vi "DatabaseView.vi"(11 "In_Database":string[][](array[string])) -> (3 "Out_Data":T1[](array[typedef]))   [LabVIEW 2020]
doc: "Na podstawie bazy danych, tworzy wizualizacjê wybieranych opcji przez w³aœciciela auta o danej tablicy rejestracyjnej."
uses:
  controls/BaseElemCluster.ctl
  controls/Car_wash_indicators.ctl
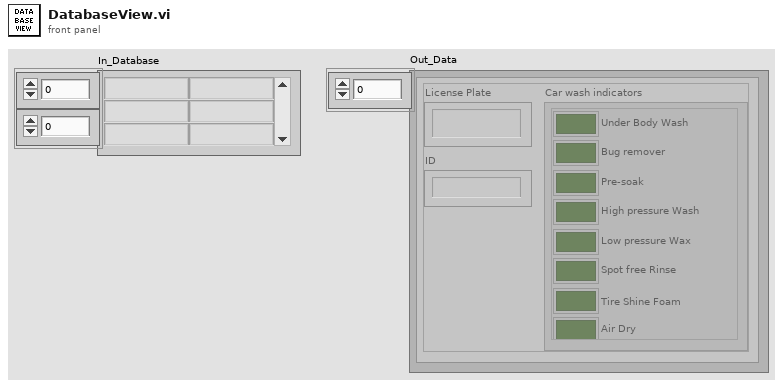
[diagram p1: front panel]
types:
  T1 = typedef "BaseElemCluster.ctl" = cluster{"ID":string, "License Plate":string, "Car wash indicators":T2}
  T2 = typedef "Car_wash_indicators.ctl" = cluster{"Under Body Wash":bool, "Bug remover":bool, "Pre-soak":bool, "High pressure Wash":bool, "Low pressure Wax":bool, "Spot free Rinse ":bool, "Tire Shine Foam ":bool, "Air Dry ":bool, "Vehicle Out of Position":bool}
  T3 = cluster{"[0]":bool, "[1]":bool, "[2]":bool, "[3]":bool, "[4]":bool, "[5]":bool, "[6]":bool, "[7]":bool, "[8]":bool}
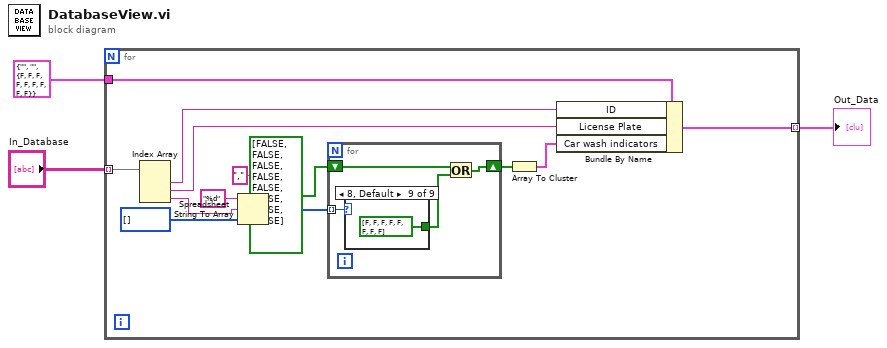
[diagram p0: block diagram]
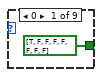
[diagram p2: hidden frame]
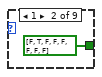
[diagram p3: hidden frame]
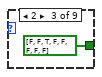
[diagram p4: hidden frame]
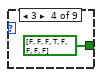
[diagram p5: hidden frame]
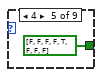
[diagram p6: hidden frame]
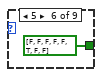
[diagram p7: hidden frame]
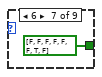
[diagram p8: hidden frame]
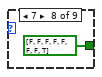
[diagram p9: hidden frame]
diagram:
  n1 = for {
    tunnel: "In_Database" -> [w15] mode=indexing
    tunnel: T1 {"ID"="", "License Plate"="", "Car wash indicators"={"Under Body Wash"=FALSE, "Bug remover"=FALSE, "Pre-soak"=FALSE, "High pressure Wash"=FALSE, "Low pressure Wax"=FALSE, "Spot free Rinse "=FALSE, "Tire Shine Foam "=FALSE, "Air Dry "=FALSE, "Vehicle Out of Position"=FALSE}} ("BaseElemCluster") -> [w16]
    tunnel: [w4] -> w1 mode=indexing
    n2 = Index Array(array=w15) -> (element #1=w14:string, element #2=w13:string, element #3=w10:string)  [unwired: 3 in]
    n3 = Spreadsheet String To Array(delimiter (Tab)=",", format string="%d", spreadsheet string=w10, array type (2D Dbl)=u8[] []) -> (array=w8:u8[])
    n4 = for {
      tunnel: w8 -> [w20] mode=indexing
      shift-right: [w17] -> w6
      shift-left: bool[] [FALSE, FALSE, FALSE, FALSE, FALSE, FALSE, FALSE, FALSE] -> [w19]
      n5 = case shown="8, Default" w20 {
        tunnel: [bool[] [TRUE, FALSE, FALSE, FALSE, FALSE, FALSE, FALSE, FALSE] bool[] [FALSE, TRUE, FALSE, FALSE, FALSE, FALSE, FALSE, FALSE] bool[] [FALSE, FALSE, TRUE, FALSE, FALSE, FALSE, FALSE, FALSE] bool[] [FALSE, FALSE, FALSE, TRUE, FALSE, FALSE, FALSE, FALSE] bool[] [FALSE, FALSE, FALSE, FALSE, TRUE, FALSE, FALSE, FALSE] bool[] [FALSE, FALSE, FALSE, FALSE, FALSE, TRUE, FALSE, FALSE] bool[] [FALSE, FALSE, FALSE, FALSE, FALSE, FALSE, TRUE, FALSE] bool[] [FALSE, FALSE, FALSE, FALSE, FALSE, FALSE, FALSE, TRUE] bool[] [FALSE, FALSE, FALSE, FALSE, FALSE, FALSE, FALSE, FALSE]] -> w18
        frame 0 {
        }
        frame 1 {
        }
        frame 2 {
        }
        frame 3 {
        }
        frame 4 {
        }
        frame 5 {
        }
        frame 6 {
        }
        frame 7 {
        }
        frame 8, Default {
        }
      }
      n6 = Or(x=w19, y=w18) -> (x .or. y?=w17:bool[])
    }
    n7 = Array To Cluster(array=w6) -> (cluster=w5:T3)
    n8 = Bundle By Name(cluster=w16, "ID"=w14, "License Plate"=w13, "Car wash indicators"=w5) -> (w4:T1)
  }
  "Out_Data" <- w1
